vi "LVClass_Image Is processed image.vi"(0 "Image in":refnum<class "Image.lvclass">, 11 "error in (no error)":errorcluster) -> (4 "Image out":refnum<class "Image.lvclass">, 6 "IsProcessedImage":bool, 15 "error out":errorcluster)   [LabVIEW 2020, in "Image.lvclass"]
doc: "Get metadata from Image object.\n\n--------------------------------------------------------------------------------\n\n<B>ImageIn </B> : Image object.\n<B>ImageOut </B> : Image object.\n<B>haso_serial_number </B> : Haso serial number.\n<B>camera_serial_number </B> : Camera serial number.\n<B>exposure_time_applied </B> : Exposure duration applied (us).\n<B>exposure_time_requested </B> : Exposure duration requested (us).\n<B>gain </B> : Applied gain (SI).\n<B>nb_summed_images </B> : Number of summed images.\n<B>is_smearing_removed </B> : Smearing_removed.\n<B>is_background_removed </B> : Background_removed.\n<B>trigger_type </B> : Trigger mode.\n<B>time_stamp </B> : Date of the acquired Image.\n<B>max_level </B> : Max level value.\n<B>comments </B> : Comments.\n<B>ErrorIn </B> : Error\n<B>ErrorOut </B> : Error\n\n--------------------------------------------------------------------------------"
uses:
  Image.lvclass
  Image.lvclass/Image.ctl
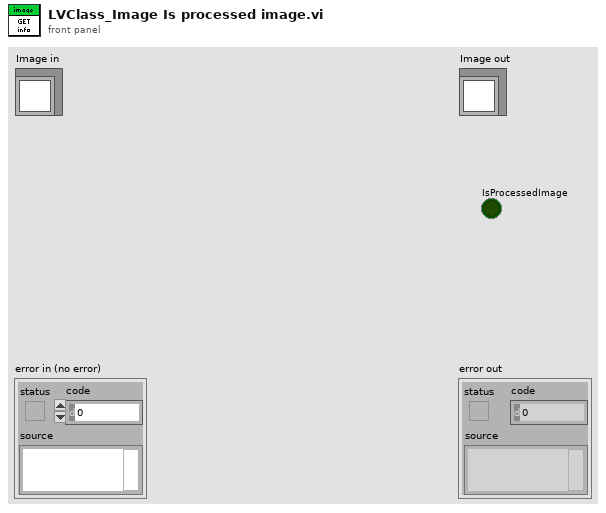
[diagram p1: front panel]
types:
  T1 = typedef "ClassID.ctl" = i64
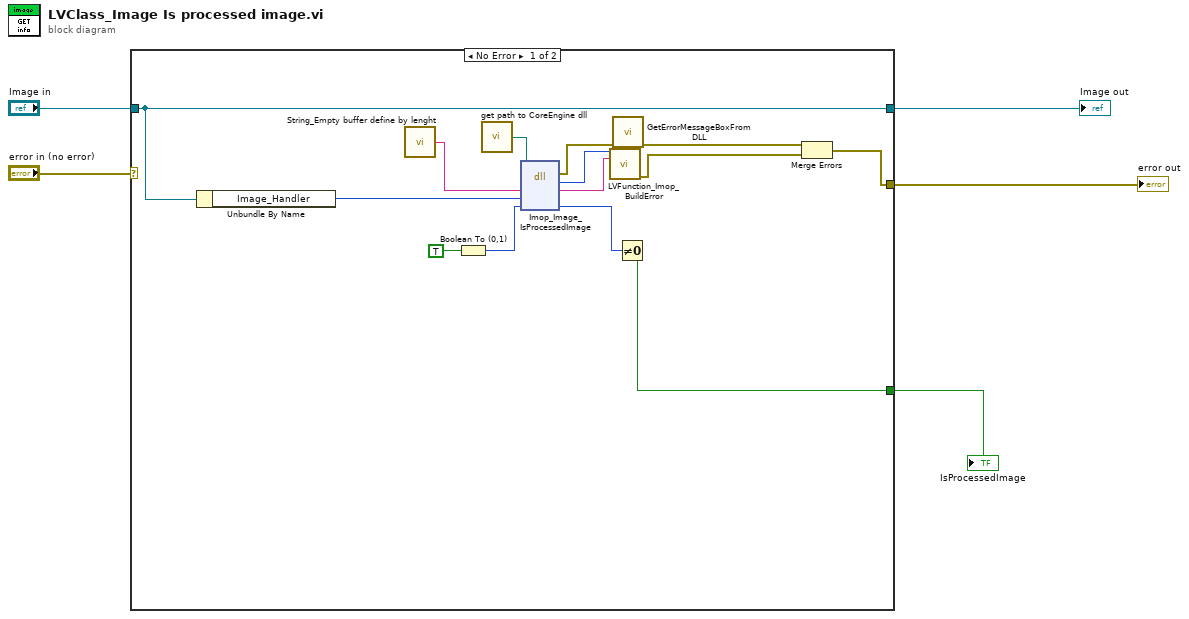
[diagram p0: block diagram]
diagram:
  n1 = case shown="No Error" "error in (no error)" {
    selector: "error in (no error)" -> [_ w21]
    tunnel: [w9 w21] -> w4
    tunnel: [w7 w20] -> w2
    tunnel: "Image in" -> [w7 w20]
    tunnel: [w6 _] -> w1
    frame No Error {
      n2 = Unbundle By Name(w7) -> ("Image_Handler"=w19:T1)
      n3 = call "String_Empty buffer define by lenght.vi"() -> ("Empty buffer"=w8:string)  [unwired: 1 in]
      n4 = Boolean To (0,1)(Boolean=TRUE) -> (0, 1=w13:i16)
      n5 = call "get path to CoreEngine dll.vi"() -> ("path to c_interface_vc100.dll"=w16:path)  [unwired: 12 in, 3 out]
      n6 = dll-call lib="D:/2_trunk/Soft_haso/ImOpCoreEngine4_LV2011/DLLs/ImopEngine4_vc100.dll" fn="Imop_Image_IsProcessedImage"(path in=w16, "message"=w8, "Image compat"=w19, "smearing_removed"=w13) -> (error out=w15:errorcluster, "return type"=w18:i32, "message"=w17:string, "smearing_removed"=w12:u8)  [unwired: 3 in, 1 out]
      n7 = call "LVFunction_Imop_BuildError.vi"("code"=w18, "String to Prepend to source (\"\")"=w17) -> ("error out"=w10:errorcluster)  [unwired: 13 in]
      n8 = call "GetErrorMessageBoxFromDLL.vi"("error IN"=w15) -> ("error OUT"=w11:errorcluster)  [unwired: 10 in]
      n9 = Not Equal To 0?(x=w12) -> (x != 0?=w6:bool)
      n10 = Merge Errors(w11, w10) -> (w9:errorcluster)
    }
    frame Error {
    }
  }
  "error out" <- w4
  "Image out" <- w2
  "IsProcessedImage" <- w1
